vi "step6 TestIfAllCornersSolved.vi"(11 "cube in 2":T1) -> (2 "all corners solved?":bool, 3 "cube in":T1)   [LabVIEW 2011]
uses:
  Typedef/cube.ctl
  Typedef/face.ctl
  Typedef/cube rotate direction.ctl
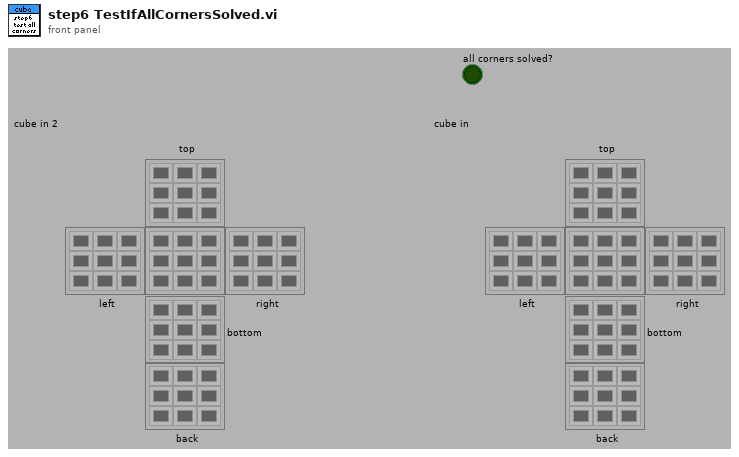
[diagram p1: front panel]
types:
  T1 = typedef "cube.ctl" = cluster{"top":T2, "left":T2, "right":T2, "bottom":T2, "back":T2, "front":T2}
  T2 = typedef "face.ctl" = u32[][]
  T3 = typedef "cube rotate direction.ctl" = enum16{"up", "down", "left", "right"}
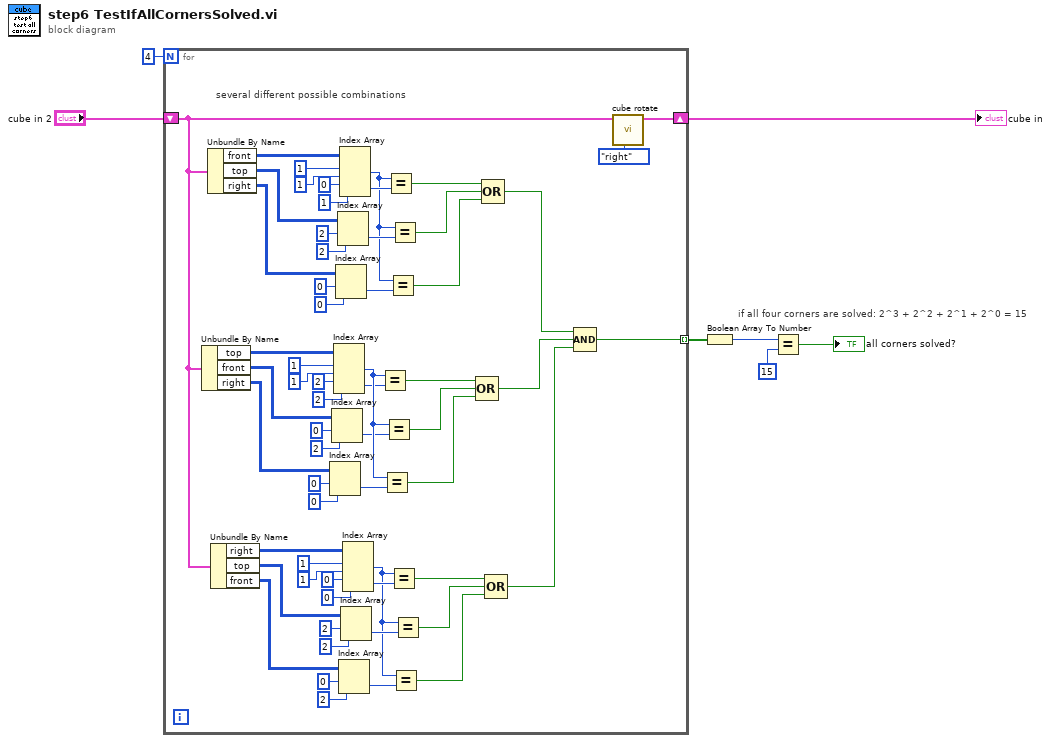
[diagram p0: block diagram]
diagram:
  # "if all four corners are solved: 2^3 + 2^2 + 2^1 + 2^0 = 15"
  n1 = for {
    N: 4 -> [_]
    shift-right: [w66] -> w7
    shift-left: "cube in 2" -> [w13]
    tunnel: [w9] -> w4 mode=indexing
    # "several different possible combinations"
    n2 = Unbundle By Name(w13) -> ("top"=w34:T2, "front"=w38:T2, "right"=w45:T2)
    n3 = Unbundle By Name(w13) -> ("front"=w65:T2, "top"=w61:T2, "right"=w54:T2)
    n4 = Unbundle By Name(w13) -> ("right"=w29:T2, "top"=w25:T2, "front"=w18:T2)
    n5 = Index Array(array=w45, index (row)=0, index (col)=0 ("disabled index (col)")) -> (element=w42:u32)
    n6 = Index Array(array=w38, index (row)=0, index (col)=2 ("disabled index (col)")) -> (element=w41:u32)
    n7 = Index Array(array=w34, index (row) #1=1 ("index (row)"), index (col) #1=1 ("disabled index (col)"), index (row) #2=2 ("index (row)"), index (col) #2=2 ("disabled index (col)")) -> (element #1=w46:u32, element #2=w37:u32)
    n8 = Index Array(array=w54, index (row)=0, index (col)=0 ("disabled index (col)")) -> (element=w57:u32)
    n9 = Index Array(array=w61, index (row)=2, index (col)=2 ("disabled index (col)")) -> (element=w58:u32)
    n10 = Index Array(array=w18, index (row)=0, index (col)=2 ("disabled index (col)")) -> (element=w21:u32)
    n11 = Index Array(array=w65, index (row) #1=1 ("index (row)"), index (col) #1=1 ("disabled index (col)"), index (row) #2=0 ("index (row)"), index (col) #2=1 ("disabled index (col)")) -> (element #1=w53:u32, element #2=w62:u32)
    n12 = Index Array(array=w25, index (row)=2, index (col)=2 ("disabled index (col)")) -> (element=w22:u32)
    n13 = Index Array(array=w29, index (row) #1=1 ("index (row)"), index (col) #1=1 ("disabled index (col)"), index (row) #2=0 ("index (row)"), index (col) #2=0 ("disabled index (col)")) -> (element #1=w17:u32, element #2=w26:u32)
    n14 = Equal?(x=w46, y=w37) -> (x = y?=w47:bool)
    n15 = Equal?(x=w46, y=w42) -> (x = y?=w49:bool)
    n16 = Equal?(x=w46, y=w41) -> (x = y?=w48:bool)
    n17 = Equal?(x=w53, y=w62) -> (x = y?=w52:bool)
    n18 = Equal?(x=w53, y=w57) -> (x = y?=w50:bool)
    n19 = Equal?(x=w17, y=w26) -> (x = y?=w16:bool)
    n20 = Equal?(x=w53, y=w58) -> (x = y?=w51:bool)
    n21 = Equal?(x=w17, y=w21) -> (x = y?=w14:bool)
    n22 = Equal?(x=w17, y=w22) -> (x = y?=w15:bool)
    n23 = Compound Arithmetic op=OR(w47, w48, w49) -> (w11:bool)
    n24 = Compound Arithmetic op=OR(w52, w51, w50) -> (w12:bool)
    n25 = Compound Arithmetic op=OR(w16, w15, w14) -> (w10:bool)
    n26 = Compound Arithmetic op=AND(w12, w11, w10) -> (w9:bool)
    n27 = call "cube rotate.vi"("cube rotation direction"=cube_rotate_direction."right", "cube in"=w13) -> ("cube out"=w66:T1)  [unwired: 8 in, 1 out]
  }
  "cube in" <- w7
  n28 = Boolean Array To Number(Boolean array=w4) -> (number=w3:u32)
  n29 = Equal?(x=w3, y=u32 15) -> (x = y?=→"all corners solved?":bool)
